vi "Pulse Generator.vi"(9 "Duty Cycle":dbl, 10 "Step size":dbl, 11 "Frequency":dbl) -> (0 "Pulse Wave":bool, 3 "Count":dbl, 4 "Max Count":dbl=100.0, 6 "Threshold count":dbl)   [LabVIEW 2018]
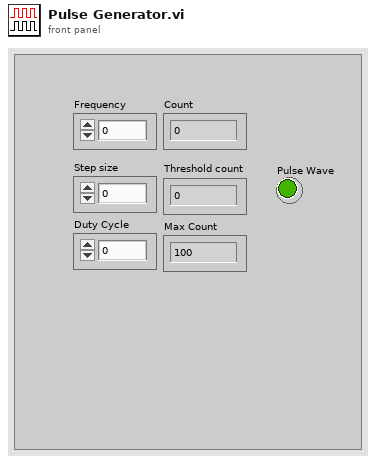
[diagram p1: front panel]
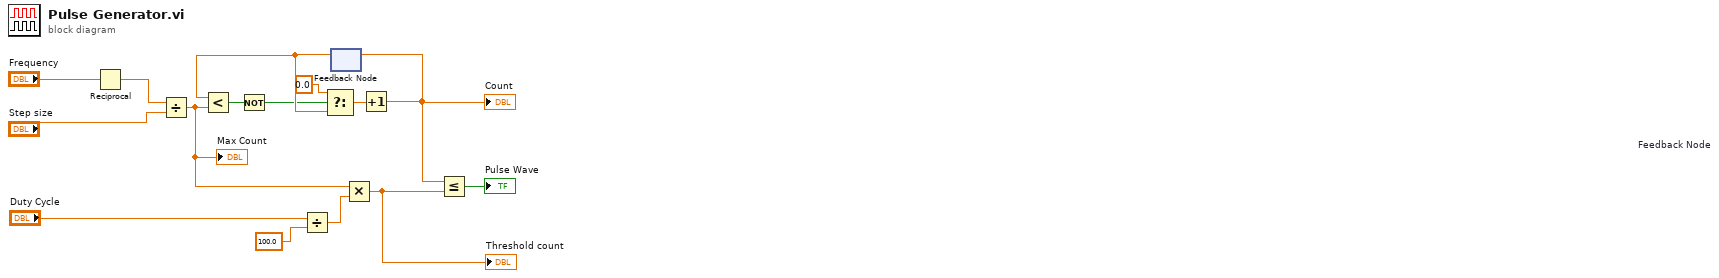
[diagram p0: block diagram]
diagram:
  n1 = Reciprocal(x="Frequency") -> (1/x=w13:dbl)
  n2 = Divide(x=w13, y="Step size") -> (x/y=w11:dbl)
  "Max Count" <- w11
  n3 = Divide ("Divide 2")(x="Duty Cycle", y=100.0) -> (x/y=w10:dbl)
  n4 = feedback #1 "Feedback Node"() -> (w5:dbl)  [unwired: 1 in]
  n5 = Less?(x=w5, y=w11) -> (x < y?=w3:bool)
  n6 = Not(x=w3) -> (.not. x?=w2:bool)
  n7 = Select(t=0.0, s=w2, f=w5) -> (s? t:f=w4:dbl)
  n8 = Multiply(x=w11, y=w10) -> (x*y=w15:dbl)
  "Threshold count" <- w15
  n9 = Increment(x=w4) -> (x+1=w12:dbl)
  "Count" <- w12
  n10 = feedback-in #1 ("2")(w12) -> ()
  n11 = Less Or Equal?(x=w12, y=w15) -> (x <= y?=→"Pulse Wave":bool)
